vi "Parse Footer.vi"(8 "error in":errorcluster, 11 "Footer":string[](array[string])) -> (0 "error out":errorcluster, 2 "DateTime":timestamp, 3 "TotalPrice":dbl format="%.2g")   [LabVIEW 2018, in "Receipt Parsing.lvlib"]
uses:
  Receipt Parsing.lvlib
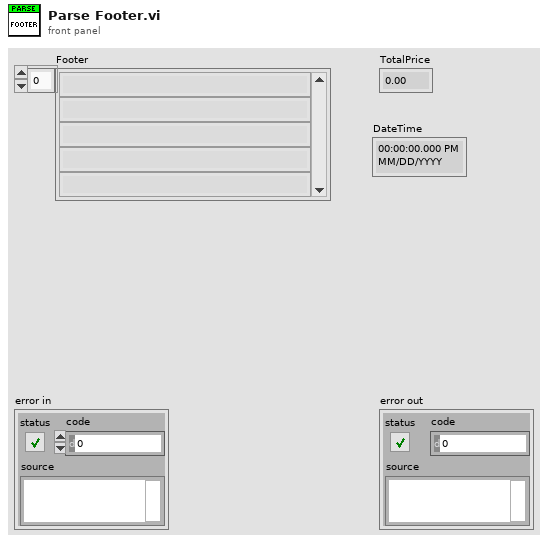
[diagram p1: front panel]
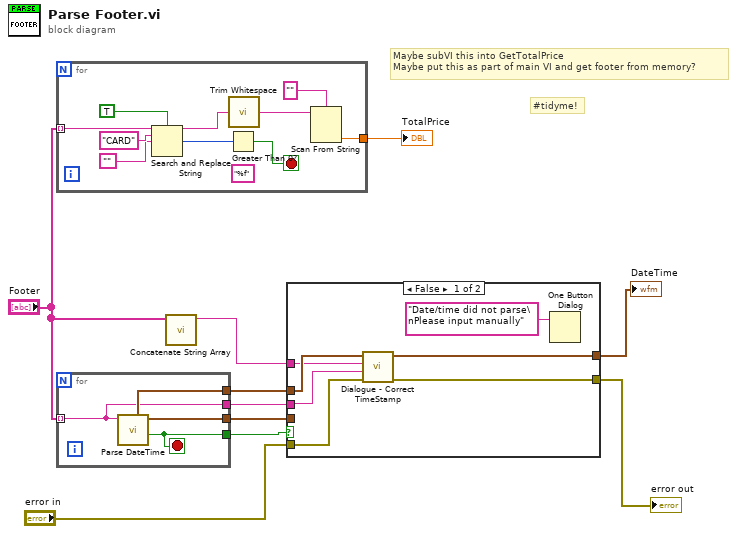
[diagram p0: block diagram]
diagram:
  # "#tidyme!"
  # "Maybe subVI this into GetTotalPrice\nMaybe put this as part of main VI and get footer from memory?"
  n1 = for {
    tunnel: "Footer" -> [w20] mode=indexing
    tunnel: [w13] -> w10
    stop <- w12 stop-if-true
    (unwired) "%f" ("format string")
    n2 = Search and Replace String(case sensitive?=TRUE ("ignore case? (F)"), input string=w20, search string="CARD", replace string="") -> (result string=w16:string, number of replacements=w11:i32)  [unwired: 4 in, 2 out]
    n3 = Greater Than 0?(x=w11) -> (x > 0?=w12:bool)
    n4 = call <vilib>:"Trim Whitespace.vi"("string"=w16) -> ("trimmed string"=w15:string)  [unwired: 1 in]
    n5 = Scan From String(format string="", input string=w15) -> (output 1=w13:dbl)  [unwired: 3 in, 3 out]
  }
  "TotalPrice" <- w10
  n6 = for {
    tunnel: "Footer" -> [w21] mode=indexing
    tunnel: [w24] -> w9
    tunnel: [w23] -> w8
    tunnel: [w22] -> w4
    tunnel: [w21] -> w3
    stop <- w23 stop-if-true
    n7 = call "Parse DateTime.vi"("Line containing datetime"=w21) -> ("Success?"=w23:bool, "time stamp"=w24:timestamp, "Partial Date (use if error)"=w22:timestamp)  [unwired: 8 in]
  }
  n8 = call "Concatenate String Array.vi"("Array"="Footer") -> ("Concatenated String"=w2:string)  [unwired: 10 in]
  n9 = case shown="False" w8 {
    tunnel: w9 -> [_ w33]
    tunnel: [w30 w33] -> w7
    tunnel: [w29 w32] -> w6
    tunnel: "error in" -> [w28 w32]
    tunnel: w4 -> [w27 _]
    tunnel: w3 -> [w26 _]
    tunnel: w2 -> [w25 _]
    frame False {
      n10 = call "Dialogue - Correct TimeStamp.vi"("error in (no error)"=w28, "Suspected Datetime"=w26, "Footer Text"=w25, "DateTime in Footer Text"=w27) -> ("error out"=w29:errorcluster, "DateTime Out"=w30:timestamp)  [unwired: 6 in]
      n11 = One Button Dialog(message="Date/time did not parse\nPlease input manually") -> ()  [unwired: 1 in, 1 out]
    }
    frame True {
    }
  }
  "error out" <- w6
  "DateTime" <- w7
